vi "dfd_Maxflat Filter Design Sort Mapping Roots.vi"(8 "error in (no error)":errorcluster, 11 "polynomial":dbl[](array[numeric]) format="%_10g") -> (0 "error out":errorcluster, 3 "roots":cdb[](array[numeric]))   [LabVIEW 2017, in "NI_DigFilter_Design.lvlib"]
doc: "Maps the roots of polynomial to z domain and sorts them by absolute value."
uses:
  <vilib>/addons/Digital Filter Design/NI_DigFilter_Design.lvlib
  <vilib>/addons/Digital Filter Design/_Misc.llb/dfd_Error Cluster From Error Code (Scalar).vi
  <vilib>/Analysis/polynomials.llb/Polynomial Roots (DBL).vi
  <vilib>/Analysis/polynomials.llb/Remove Zero Coefficients (DBL).vi
  <vilib>/Analysis/NI_AALPro.lvlib
  <vilib>/addons/Digital Filter Design/NI_DigFilterLicensed.lvlib
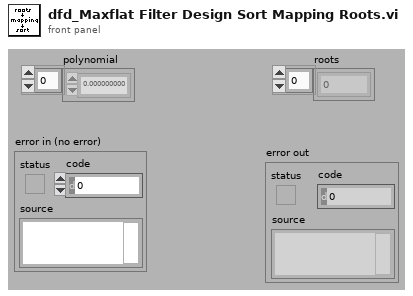
[diagram p1: front panel]
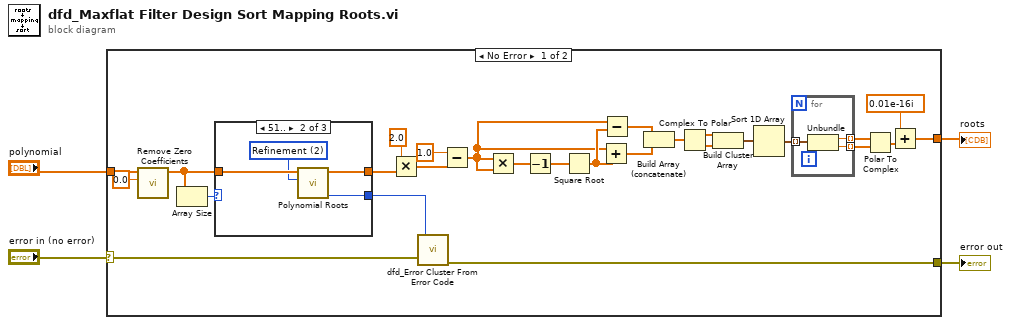
[diagram p0: block diagram]
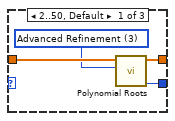
[diagram p2: hidden frame]
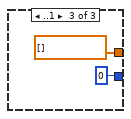
[diagram p3: hidden frame]
diagram:
  n1 = case shown="No Error" "error in (no error)" {
    selector: "error in (no error)" -> [w6 w45]
    tunnel: "polynomial" -> [w15 _]
    tunnel: [w13 w45] -> w3
    tunnel: [w10 _] -> w2
    frame No Error {
      n2 = call-poly <vilib>:"Remove Zero Coefficients.vi"("threshold"=0.0, "P(x) In"=w15) -> ("P(x) Out"=w8:dbl[])  [unwired: 1 in, 8 out]
      n3 = Array Size(array=w8) -> (size(s)=w5:i32)
      n4 = case shown="51.." w5 {
        tunnel: [w35 w39 cdb[] [] ("Complex Pair Roots")] -> w17
        tunnel: w8 -> [w33 w37 _]
        tunnel: [w34 w38 0 ("error")] -> w14
        frame 2..50, Default {
          w32 = u16 3 items=["General", "Simple Classification", "Refinement", "Advanced Refinement"] ("option")
          n5 = call-poly <vilib>:"Polynomial Roots.vi"("option"=w32, "P(x)"=w33) -> ("error"=w34:i32, "Roots"=w35:cdb[])  [unwired: 1 in, 7 out]
        }
        frame 51.. {
          w36 = u16 2 items=["General", "Simple Classification", "Refinement", "Advanced Refinement"] ("option")
          n6 = call-poly <vilib>:"Polynomial Roots.vi"("option"=w36, "P(x)"=w37) -> ("error"=w38:i32, "Roots"=w39:cdb[])  [unwired: 1 in, 7 out]
        }
        frame ..1 {
        }
      }
      n7 = Multiply(x=2.0, y=w17) -> (x*y=w19:cdb[])
      n8 = call-poly <vilib>:"dfd_Error Cluster From Error Code.vi"("error in (no error)"=w6, "error code (0)"=w14) -> ("error out"=w13:errorcluster)  [unwired: 9 out]
      n9 = Subtract(x=1.0, y=w19) -> (x-y=w11:cdb[])
      n10 = Multiply(x=w11, y=w11) -> (x*y=w12:cdb[])
      n11 = Decrement(x=w12) -> (x-1=w21:cdb[])
      n12 = Square Root(x=w21) -> (sqrt(x)=w22:cdb[])
      n13 = Add(x=w11, y=w22) -> (x+y=w24:cdb[])
      n14 = Subtract(x=w11, y=w22) -> (x-y=w23:cdb[])
      n15 = Build Array (concatenate)(w23, w24) -> (w25:cdb[])
      n16 = Complex To Polar(r * e^(i*theta)=w25) -> (r=w26:dbl[], theta=w27:dbl[])
      n17 = Build Cluster Array(w26, w27) -> (w28:cluster{dbl, dbl}[])
      n18 = Sort 1D Array(array=w28) -> (sorted array=w29:cluster{dbl, dbl}[])
      n19 = for {
        tunnel: w29 -> [w44] mode=indexing
        tunnel: [w43] -> w30 mode=indexing
        tunnel: [w42] -> w31 mode=indexing
        n20 = Unbundle(w44) -> (w43:dbl, w42:dbl)
      }
      n21 = Polar To Complex(1:w31, 2:w30) -> (0:w16:cdb[])
      n22 = Add(x=cdb 0.0+1e-16i, y=w16) -> (x+y=w10:cdb[])
    }
    frame Error {
    }
  }
  "error out" <- w3
  "roots" <- w2
